vi "readTelemetryMirrorForceData.vi"(8 "error in (no error)":errorcluster, 10 "Parser":refnum<class "U8ArrayParserAutoIndexing.lvclass">, 11 "M1M3SAL in":refnum<class "M1M3SAL.lvclass">) -> (0 "error out":errorcluster, 2 "EventSummaryState":variant, 3 "M1M3SAL out":refnum<class "M1M3SAL.lvclass">)   [LabVIEW 2016, in "M1M3SupportCommunicator.lvlib" / "M1M3SAL.lvclass"]
uses:
  M1M3SAL.lvclass
  Common_RT_Utilities/U8ArrayParserAutoIndexing/U8ArrayParserAutoIndexing.lvclass
  DataTypes/Topics/TelemetryMirrorForceData.ctl
  DataTypes/Topics/Parts/Timestamp.ctl
  DataTypes/Topics/M1M3SupportTopics.lvlib
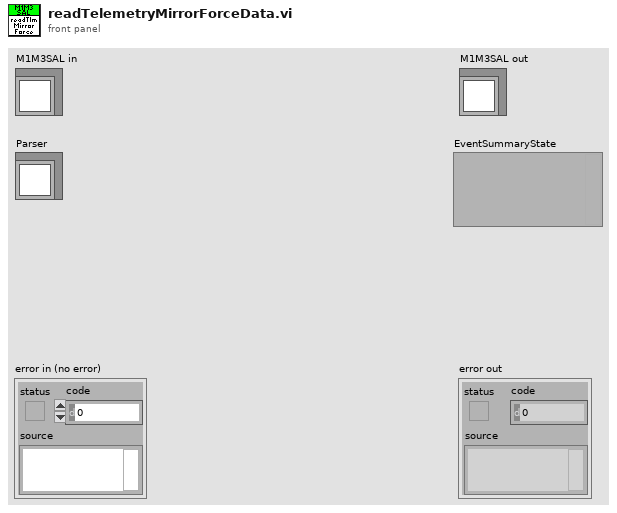
[diagram p1: front panel]
types:
  T1 = typedef "M1M3SupportTopics.lvlib/TelemetryMirrorForceData.ctl" = cluster{"Timestamp":T2, "Fx":dbl, "Fy":dbl, "Fz":dbl, "Mx":dbl, "My":dbl, "Mz":dbl}
  T2 = typedef "M1M3SupportTopics.lvlib/Timestamp.ctl" = dbl
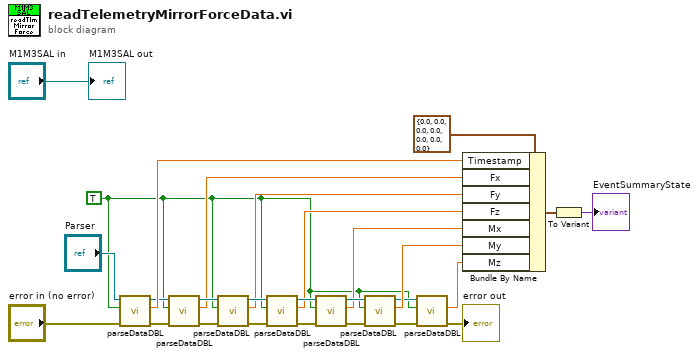
[diagram p0: block diagram]
diagram:
  w1 = TRUE ("OverrideSwapBytes")
  n1 = call "parseDataDBL.vi"("error in (no error)"="error in (no error)", "OverrideSwapBytes"=w1, "U8ArrayParserAutoIndexing in"="Parser") -> ("error out"=w12:errorcluster, "Data"=w22:dbl, "U8ArrayParserAutoIndexing out"=w14:refnum<class "U8ArrayParserAutoIndexing.lvclass">)  [unwired: 6 in]
  n2 = call "parseDataDBL.vi"("error in (no error)"=w12, "OverrideSwapBytes"=w1, "U8ArrayParserAutoIndexing in"=w14) -> ("error out"=w11:errorcluster, "Data"=w10:dbl, "U8ArrayParserAutoIndexing out"=w13:refnum<class "U8ArrayParserAutoIndexing.lvclass">)  [unwired: 6 in]
  n3 = call "parseDataDBL.vi"("error in (no error)"=w11, "OverrideSwapBytes"=w1, "U8ArrayParserAutoIndexing in"=w13) -> ("error out"=w20:errorcluster, "Data"=w9:dbl, "U8ArrayParserAutoIndexing out"=w19:refnum<class "U8ArrayParserAutoIndexing.lvclass">)  [unwired: 6 in]
  n4 = call "parseDataDBL.vi"("error in (no error)"=w20, "OverrideSwapBytes"=w1, "U8ArrayParserAutoIndexing in"=w19) -> ("error out"=w18:errorcluster, "Data"=w8:dbl, "U8ArrayParserAutoIndexing out"=w17:refnum<class "U8ArrayParserAutoIndexing.lvclass">)  [unwired: 6 in]
  n5 = call "parseDataDBL.vi"("error in (no error)"=w18, "OverrideSwapBytes"=w1, "U8ArrayParserAutoIndexing in"=w17) -> ("error out"=w16:errorcluster, "Data"=w7:dbl, "U8ArrayParserAutoIndexing out"=w15:refnum<class "U8ArrayParserAutoIndexing.lvclass">)  [unwired: 6 in]
  n6 = call "parseDataDBL.vi"("error in (no error)"=w16, "OverrideSwapBytes"=w1, "U8ArrayParserAutoIndexing in"=w15) -> ("error out"=w4:errorcluster, "Data"=w6:dbl, "U8ArrayParserAutoIndexing out"=w5:refnum<class "U8ArrayParserAutoIndexing.lvclass">)  [unwired: 6 in]
  n7 = call "parseDataDBL.vi"("error in (no error)"=w4, "OverrideSwapBytes"=w1, "U8ArrayParserAutoIndexing in"=w5) -> ("error out"=→"error out":errorcluster, "Data"=w2:dbl)  [unwired: 6 in, 1 out]
  n8 = Bundle By Name(cluster=T1 {"Timestamp"=0.0, "Fx"=0.0, "Fy"=0.0, "Fz"=0.0, "Mx"=0.0, "My"=0.0, "Mz"=0.0} ("TelemetryMirrorForceData"), "Timestamp"=w22, "Fx"=w10, "Fy"=w9, "Fz"=w8, "Mx"=w7, "My"=w6, "Mz"=w2) -> (w26:T1)
  n9 = To Variant(anything=w26) -> (Variant=→"EventSummaryState":variant)
  "M1M3SAL out" <- "M1M3SAL in"
